vi "Template - Power Meter Acquire Measurement.vi"() -> ()   [LabVIEW 2020]
doc: "This example shows how to acquire a power measurement using the VIs of the driver."
uses:
  <instrlib>/_Template - Power Meter/Template - Power Meter.lvlib
panel:
  in  "Timeout (10000 ms)":u32=10000
  out "Measurement":dbl
  in  "VISA resource name":refnum<visa-resource-name>
  # "(c) 2014 <Enter Company Name Here>.  ALL RIGHTS RESERVED."
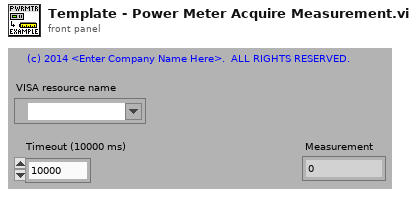
[diagram p1: front panel]
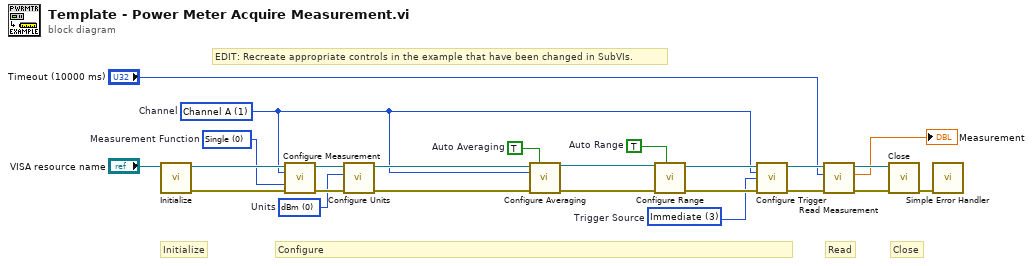
[diagram p0: block diagram]
diagram:
  w1 = u16 3 items=["Bus", "External", "Hold", "Immediate", "Internal A", "Internal B"]  # Trigger Source
  w4 = u16 0 items=["Single", "Difference", "Ratio"]  # Measurement Function
  w2 = u16 0 items=["dBm", "W"]  # Units
  w5 = TRUE  # Auto Averaging
  w6 = TRUE  # Auto Range
  w3 = u16 1 items=["Channel A"=1, "Channel B"=2]  # Channel
  # "EDIT: Recreate appropriate controls in the example that have been changed in SubVIs."
  # "Close"
  # "Read"
  # "Configure"
  # "Initialize"
  n1 = call <instrlib>:"Initialize.vi"("VISA resource name"="VISA resource name") -> ("error out"=w24:errorcluster, "VISA resource name out"=w23:refnum<visa-resource-name>)  [unwired: 9 in]
  n2 = call <instrlib>:"Configure Measurement.vi"("VISA resource name"=w23, "First Channel (1: Channel A)"=w3, "Measurement Function (0: Single)"=w4, "error in (no error)"=w24) -> ("VISA resource name out"=w22:refnum<visa-resource-name>, "error out"=w21:errorcluster)  [unwired: 10 in]
  n3 = call <instrlib>:"Configure Units.vi"("error in (no error)"=w21, "Units (0: dBm)"=w2, "VISA resource name"=w22) -> ("error out"=w20:errorcluster, "VISA resource name out"=w19:refnum<visa-resource-name>)  [unwired: 7 in]
  n4 = call <instrlib>:"Configure Averaging.vi"("VISA resource name"=w19, "Auto Averaging (T: Enable)"=w5, "Channel (1: Channel A)"=w3, "error in (no error)"=w20) -> ("VISA resource name out"=w17:refnum<visa-resource-name>, "error out"=w18:errorcluster)  [unwired: 10 in]
  n5 = call <instrlib>:"Configure Range.vi"("Auto Range (T: Enable)"=w6, "error in (no error)"=w18, "VISA resource name"=w17) -> ("error out"=w16:errorcluster, "VISA resource name out"=w15:refnum<visa-resource-name>)  [unwired: 7 in]
  n6 = call <instrlib>:"Configure Trigger.vi"("VISA resource name"=w15, "Channel (1: Channel A)"=w3, "Trigger Source (3: Immediate)"=w1, "error in (no error)"=w16) -> ("VISA resource name out"=w14:refnum<visa-resource-name>, "error out"=w13:errorcluster)  [unwired: 10 in]
  n7 = call <instrlib>:"Read Measurement.vi"("error in (no error)"=w13, "Timeout (10000 ms)"="Timeout (10000 ms)", "VISA resource name"=w14) -> ("error out"=w12:errorcluster, "Measurement"=→"Measurement":dbl, "VISA resource name out"=w11:refnum<visa-resource-name>)  [unwired: 6 in]
  n8 = call <instrlib>:"Close.vi"("error in (no error)"=w12, "VISA resource name"=w11) -> ("error out"=w9:errorcluster)  [unwired: 9 in]
  n9 = call <vilib>:"Simple Error Handler.vi"("error in (no error)"=w9) -> ()  [unwired: 4 in, 5 out]
